vi "CANFrame_DataExtract.vi"(11 "CANDATA":u8[](array[numeric])) -> (3 "Extracted Data":string[](array[string]))   [LabVIEW 2026]
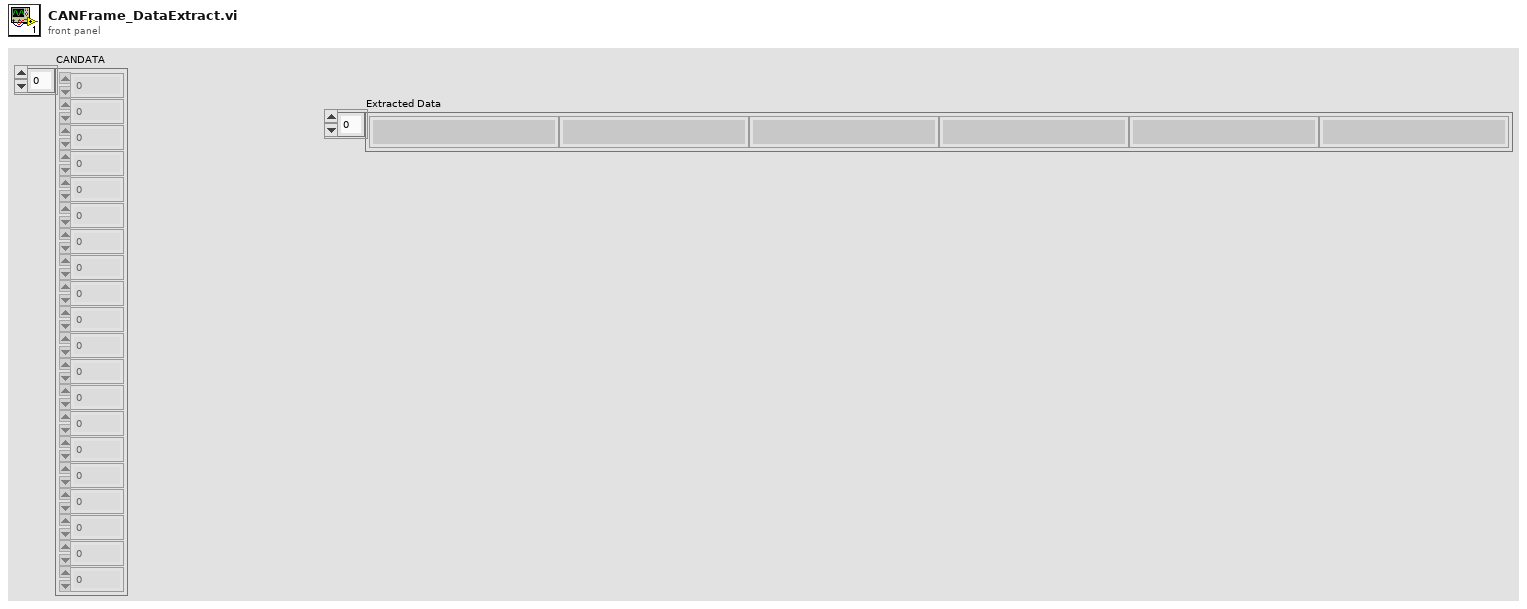
[diagram p1: front panel]
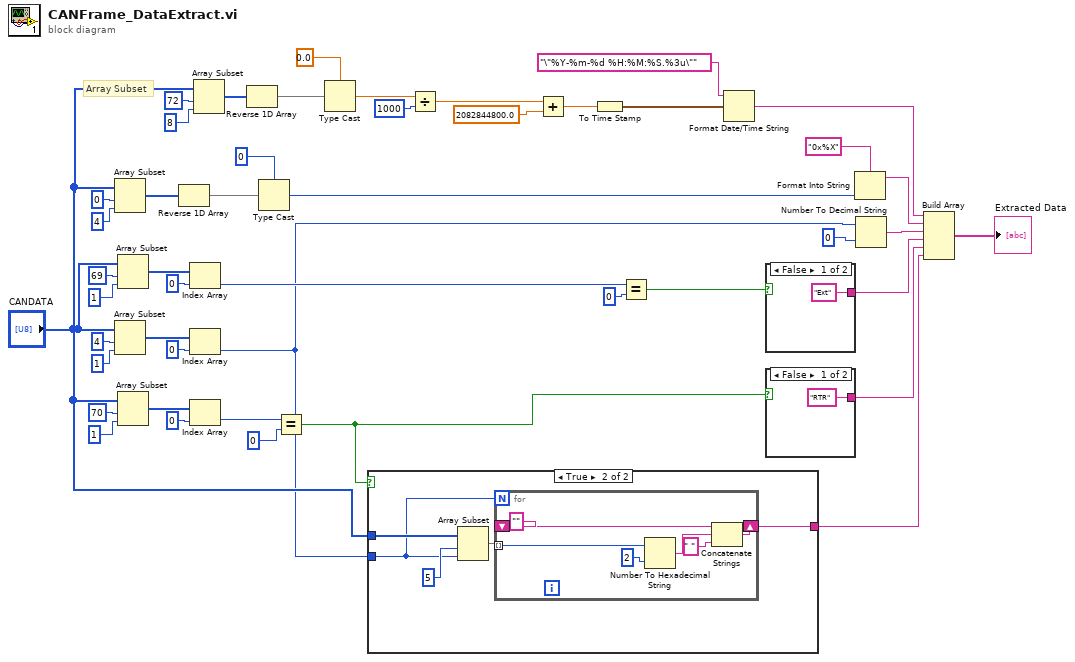
[diagram p0: block diagram]
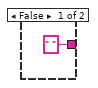
[diagram p2: hidden frame]
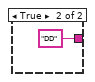
[diagram p3: hidden frame]
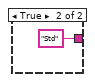
[diagram p4: hidden frame]
diagram:
  # "Array Subset"
  n1 = Array Subset(array="CANDATA", index=0, length=4) -> (w44:u8[])
  n2 = Array Subset(array="CANDATA", index=4, length=1) -> (w40:u8[])
  n3 = Array Subset(array="CANDATA", index=69, length=1) -> (w32:u8[])
  n4 = Array Subset(array="CANDATA", index=70, length=1) -> (w31:u8[])
  n5 = Reverse 1D Array(array=w44) -> (reversed array=w43:u8[])
  n6 = Index Array(array=w32, index=0) -> (element=w20:u8)
  n7 = Index Array(array=w40, index=0) -> (element=w3:u8)
  n8 = Index Array(array=w31, index=0) -> (element=w5:u8)
  n9 = Array Subset(array="CANDATA", index=72, length=8) -> (w28:u8[])
  n10 = Reverse 1D Array(array=w28) -> (reversed array=w27:u8[])
  n11 = Type Cast(type=u32 0, x=w43) -> (*(type *) &x=w25:u32)
  n12 = Equal?(x=w5, y=0) -> (x = y?=w4:bool)
  n13 = Type Cast(type=0.0, x=w27) -> (*(type *) &x=w9:dbl)
  n14 = case shown="True" w4 {
    tunnel: "CANDATA" -> [_ w51]
    tunnel: w3 -> [_ w49]
    tunnel: [" " w50] -> w6
    frame False {
    }
    frame True {
      n15 = Array Subset(array=w51, index=5, length=w49) -> (w52:u8[])
      n16 = for {
        N: w49 -> [_]
        tunnel: w52 -> [w59] mode=indexing
        shift-right: [w56] -> w50
        shift-left: "" -> [w58]
        n17 = Number To Hexadecimal String(1:2, 2:w59) -> (0:w57:string)
        n18 = Concatenate Strings(w58, w57, " " ("string")) -> (w56:string)
      }
    }
  }
  n19 = Divide(x=w9, y=1000) -> (x/y=w10:dbl)
  n20 = Add(x=w10, y=2082844800.0) -> (x+y=w13:dbl)
  n21 = To Time Stamp(1:w13) -> (0:w12:timestamp)
  n22 = Equal?(x=w20, y=u8 0) -> (x = y?=w21:bool)
  n23 = Format Date/Time String(time format string (%c)="\"%Y-%m-%d %H:%M:%S.%3u\"", seconds (now)=w12) -> (date/time string=w8:string)  [unwired: 1 in]
  n24 = case shown="False" w21 {
    tunnel: ["Ext" "Std"] -> w18
    frame False {
    }
    frame True {
    }
  }
  n25 = case shown="False" w4 {
    tunnel: ["RTR" "DD"] -> w16
    frame False {
    }
    frame True {
    }
  }
  n26 = Format Into String(format string="0x%X", w25) -> (resulting string=w23:string)  [unwired: 2 in, 1 out]
  n27 = Number To Decimal String(number=w3, width (-)=0) -> (decimal integer string=w1:string)
  n28 = Build Array "Build Array"(w8, w23, w1, w18, w16, w6) -> (→"Extracted Data":string[])
